vi "Calculate cursors' distances.vi"(8 "error in (no error)":errorcluster, 11 "XY Graph":refnum<vi>) -> (0 "error out":errorcluster, 2 "All cursors' dist.":T2)   [LabVIEW 2014]
uses:
  Controls/dist. between cursors.ctl
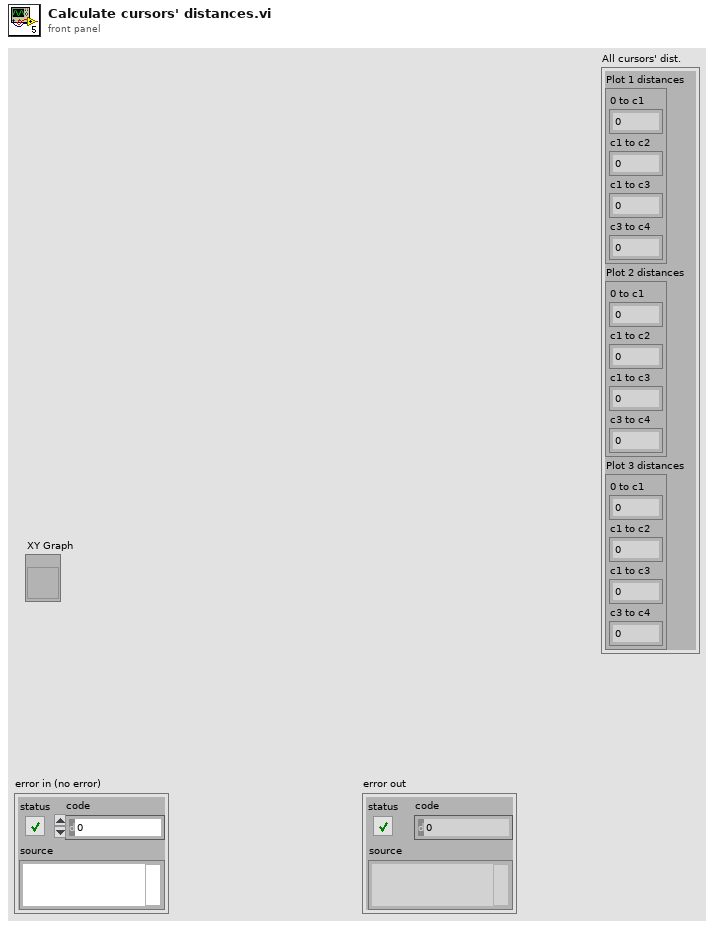
[diagram p1: front panel]
types:
  T1 = typedef "dist. between cursors.ctl" = cluster{"0 to c1":dbl, "c1 to c2":dbl, "c1 to c3":dbl, "c3 to c4":dbl}
  T2 = cluster{"Plot 1 distances":T1, "Plot 2 distances":T1, "Plot 3 distances":T1}
  T3 = typedef "LVCursorListTypeDef.ctl" = cluster{"Name":string, "Color":u32, "Style":u8, "Point Style":u8, "Name Visible":bool, "Allow Drag":bool, "Cursor Mode":u32, "Plot":i32, "Index":i32, "Position":cluster{"X":dbl, "Y":dbl}, "X Scale":u32, "Y Scale":u32, "Watch Plots":i32[], "Watch All Plots":bool, "Plot Area":i32, "Label Offset":cluster{"X":dbl, "Y":dbl}}[]
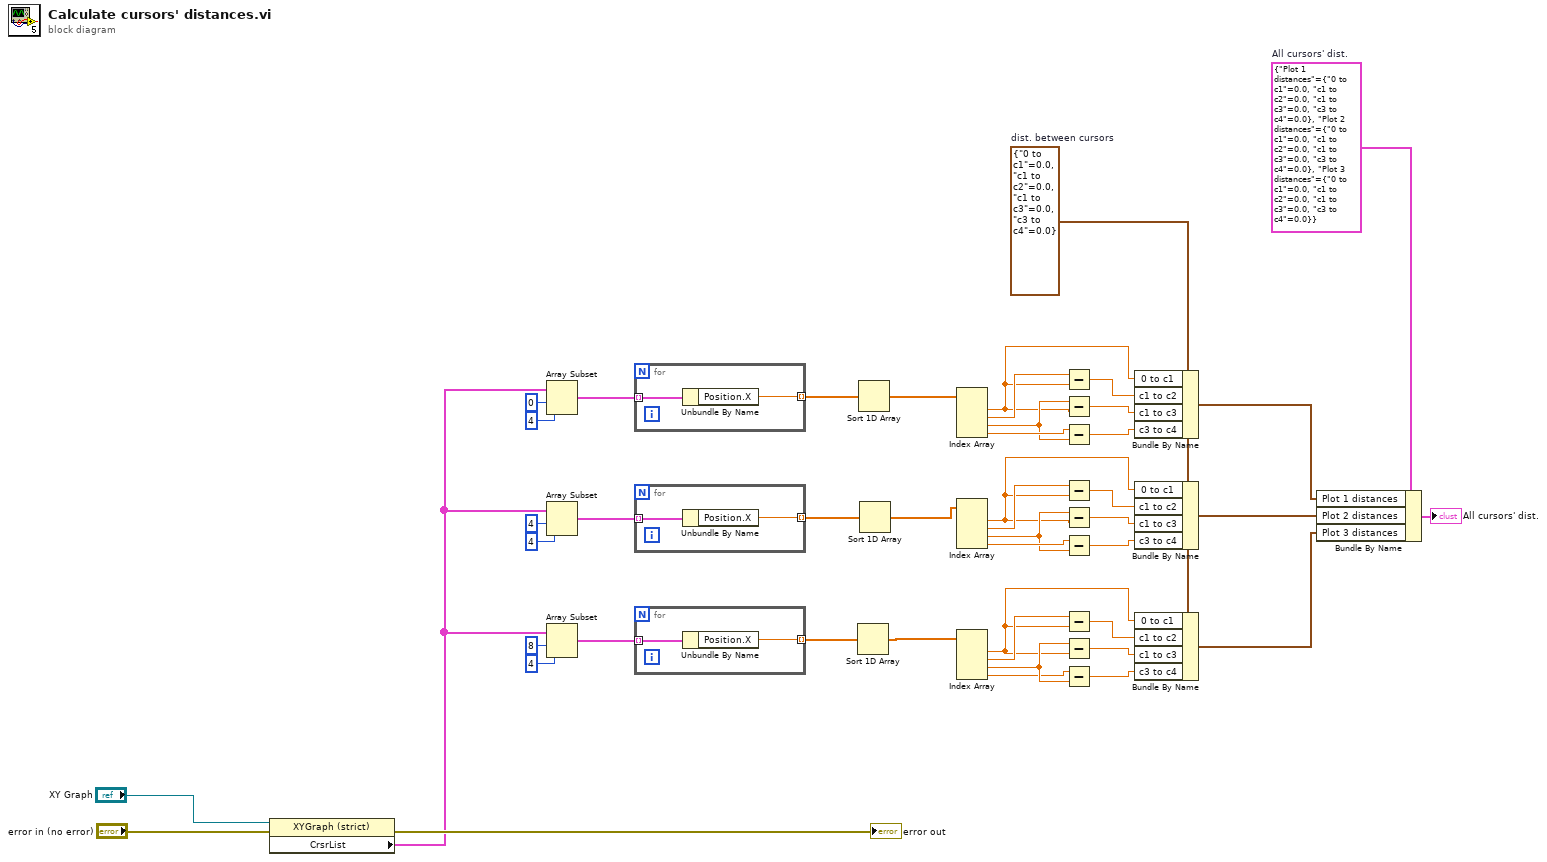
[diagram p0: block diagram]
diagram:
  w8 = T2 {"Plot 1 distances"={"0 to c1"=0.0, "c1 to c2"=0.0, "c1 to c3"=0.0, "c3 to c4"=0.0}, "Plot 2 distances"={"0 to c1"=0.0, "c1 to c2"=0.0, "c1 to c3"=0.0, "c3 to c4"=0.0}, "Plot 3 distances"={"0 to c1"=0.0, "c1 to c2"=0.0, "c1 to c3"=0.0, "c3 to c4"=0.0}}  # All cursors' dist.
  w9 = T1 {"0 to c1"=0.0, "c1 to c2"=0.0, "c1 to c3"=0.0, "c3 to c4"=0.0}  # dist. between cursors
  n1 = property class="XYGraph (strict)"(reference="XY Graph", error in="error in (no error)") -> (error out=→"error out":errorcluster, "CrsrList"=w34:T3)  [unwired: 1 out]
  n2 = Array Subset(array=w34, index=0, length=4) -> (w43:T3)
  n3 = Array Subset(array=w34, index=4, length=4) -> (w40:T3)
  n4 = Array Subset(array=w34, index=8, length=4) -> (w35:T3)
  n5 = for {
    tunnel: w43 -> [w48] mode=indexing
    tunnel: [w47] -> w33 mode=indexing
    n6 = Unbundle By Name(w48) -> ("Position.X"=w47:dbl)
  }
  n7 = for {
    tunnel: w40 -> [w50] mode=indexing
    tunnel: [w49] -> w32 mode=indexing
    n8 = Unbundle By Name(w50) -> ("Position.X"=w49:dbl)
  }
  n9 = for {
    tunnel: w35 -> [w52] mode=indexing
    tunnel: [w51] -> w31 mode=indexing
    n10 = Unbundle By Name(w52) -> ("Position.X"=w51:dbl)
  }
  n11 = Sort 1D Array(array=w31) -> (sorted array=w10:dbl[])
  n12 = Sort 1D Array(array=w33) -> (sorted array=w30:dbl[])
  n13 = Sort 1D Array(array=w32) -> (sorted array=w17:dbl[])
  n14 = Index Array(array=w30) -> (element #1=w4:dbl, element #2=w27:dbl, element #3=w28:dbl, element #4=w29:dbl)  [unwired: 4 in]
  n15 = Index Array(array=w17) -> (element #1=w3:dbl, element #2=w21:dbl, element #3=w22:dbl, element #4=w23:dbl)  [unwired: 4 in]
  n16 = Index Array(array=w10) -> (element #1=w2:dbl, element #2=w13:dbl, element #3=w12:dbl, element #4=w11:dbl)  [unwired: 4 in]
  n17 = Subtract(x=w27, y=w4) -> (x-y=w26:dbl)
  n18 = Subtract(x=w28, y=w4) -> (x-y=w25:dbl)
  n19 = Subtract(x=w29, y=w28) -> (x-y=w24:dbl)
  n20 = Subtract(x=w21, y=w3) -> (x-y=w20:dbl)
  n21 = Subtract(x=w22, y=w3) -> (x-y=w19:dbl)
  n22 = Subtract(x=w23, y=w22) -> (x-y=w18:dbl)
  n23 = Subtract(x=w13, y=w2) -> (x-y=w14:dbl)
  n24 = Subtract(x=w12, y=w2) -> (x-y=w15:dbl)
  n25 = Subtract(x=w11, y=w12) -> (x-y=w16:dbl)
  n26 = Bundle By Name(cluster=w9, "0 to c1"=w4, "c1 to c2"=w26, "c1 to c3"=w25, "c3 to c4"=w24) -> (w7:T1)
  n27 = Bundle By Name(cluster=w9, "0 to c1"=w3, "c1 to c2"=w20, "c1 to c3"=w19, "c3 to c4"=w18) -> (w6:T1)
  n28 = Bundle By Name(cluster=w9, "0 to c1"=w2, "c1 to c2"=w14, "c1 to c3"=w15, "c3 to c4"=w16) -> (w5:T1)
  n29 = Bundle By Name(cluster=w8, "Plot 1 distances"=w7, "Plot 2 distances"=w6, "Plot 3 distances"=w5) -> (→"All cursors' dist.":T2)
